vi "Test UDP Send.vi"() -> ()   [LabVIEW 2014]
doc: "Creates a write-only UDP multicast session and sends data to the specified port."
uses:
  <vilib>/Utility/tcp.llb/UDP Multicast Write-Only Open.vi
panel:
  in  "data in":string
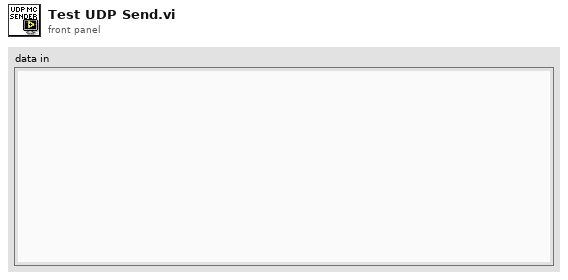
[diagram p1: front panel]
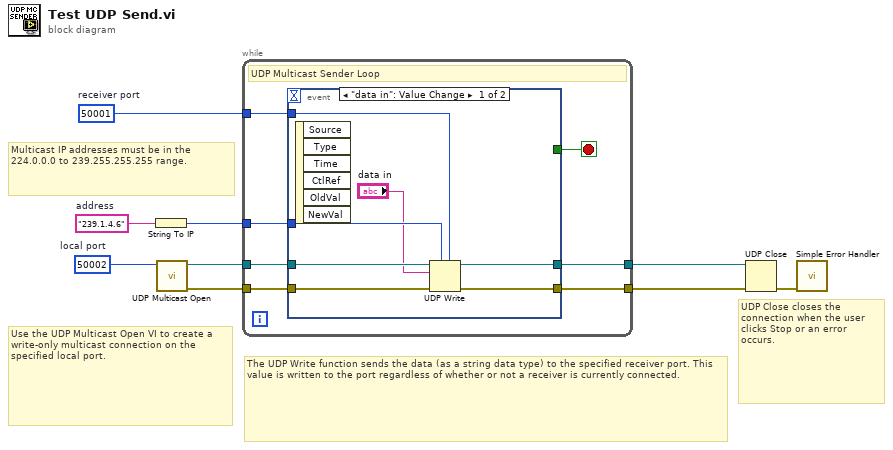
[diagram p0: block diagram]
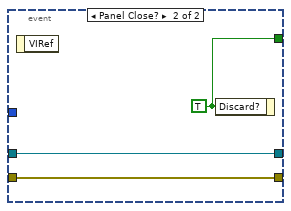
[diagram p2: hidden frame]
diagram:
  w1 = u16 50001  # receiver port
  w2 = u16 50002  # local port
  w7 = "239.1.4.6"  # address
  # "UDP Close closes the connection when the user clicks Stop or an error occurs."
  # "Multicast IP addresses must be in the 224.0.0.0 to 239.255.255.255 range."
  # "The UDP Write function sends the data (as a string data type) to the specified receiver port. This value is written to the port regardless of whether or not a receiver is currently connected."
  # "Use the UDP Multicast Open VI to create a write-only multicast connection on the specified local port."
  n1 = String To IP(1:w7) -> (0:w5:u32)
  n2 = call-poly <vilib>:"UDP Multicast Open.vi"("port"=w2) -> ("error out"=w3:errorcluster, "connection ID"=w4:refnum<k16>)  [unwired: 9 in]
  n3 = while {
    tunnel: [w13] -> w8
    tunnel: w4 -> [w16]
    tunnel: w3 -> [w15]
    tunnel: [w14] -> w9
    tunnel: w5 -> [w12]
    tunnel: w1 -> [w11]
    stop <- w10 stop-if-true
    # "UDP Multicast Sender Loop"
    n4 = event shown="[0] \"data in\": Value Change" {
      selector: _ -> [_ _]
      dyn-events: _ -> [_ _]
      timeout: _ -> [_ _]
      tunnel: w16 -> [w23 w25]
      tunnel: w15 -> [w22 w24]
      tunnel: [w21 w25] -> w14
      tunnel: [w20 w24] -> w13
      tunnel: w12 -> [w19 _]
      tunnel: w11 -> [w18 _]
      tunnel: [_ w26] -> w10
      event "data in": Value Change {
        n5 = event-data() -> ()  [unwired: 1 in, 6 out]
        n6 = UDP Write(address=w19, port or service name=w18, connection ID=w23, data in="data in", 8:w22) -> (error out=w20:errorcluster, 3:w21:refnum<k16>)  [unwired: 1 in]
      }
      event Panel Close? {
        w26 = TRUE ("Discard?")
        n7 = event-data() -> ()  [unwired: 1 in, 1 out]
        n8 = event-data("Discard?"=w26) -> ()  [unwired: 1 in, 1 out]
      }
    }
  }
  n9 = UDP Close(connection ID=w9, 8:w8) -> (error out=w6:errorcluster)  [unwired: 1 out]
  n10 = call <vilib>:"Simple Error Handler.vi"("error in (no error)"=w6) -> ()  [unwired: 4 in, 5 out]
